vi "3DS Scene Mode.vi"(8 "error in (no error)":errorcluster, 10 "Draw Style:Mode":T1(ring), 11 "SceneObject in":refnum<vi>) -> (0 "error out":errorcluster, 3 "SceneObject out":refnum<vi>)   [LabVIEW 2026, in "3D utilities.lvlib"]
uses:
  3D utilities.lvlib
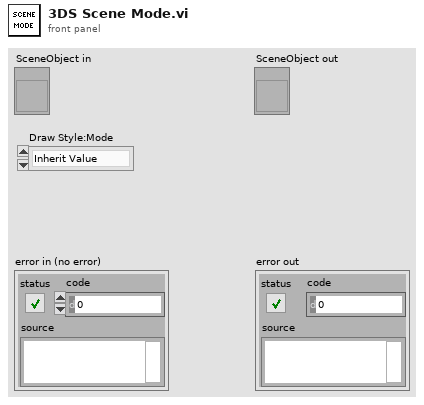
[diagram p1: front panel]
types:
  T1 = enum16{"Inherit Value", "Points", "Wireframe", "Polygons"}
  T2 = enum16{"Inherit Value", "No Culling", "Cull Back Face", "Cull Front Face", "Cull Both Faces"}
  T3 = enum16{"Zero", "One", "Destination Color", "One Minus Destination Color", "Source Alpha", "One Minus Source Alpha", "Destination Alpha", "One Minus Destination Alpha", "Source Alpha Saturate"}
  T4 = enum16{"Zero", "One", "Source Color", "One Minus Source Color", "Source Alpha", "One Minus Source Alpha", "Destination Alpha", "One Minus Destination Alpha"}
  T5 = enum16{"Normal Bin", "Opaque Bin", "Transparent Bin"}
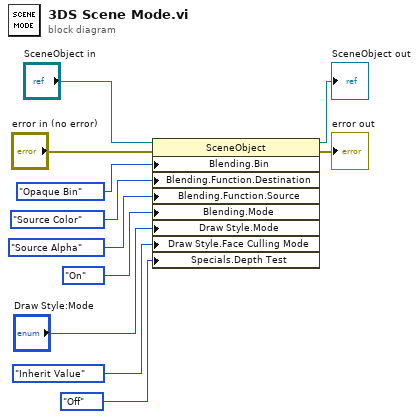
[diagram p0: block diagram]
diagram:
  n1 = property class="SceneObject"(reference="SceneObject in", error in="error in (no error)", "Blending.Bin"=T5."Opaque Bin" ("Blending:Bin"), "Blending.Function.Destination"=T4."Source Color" ("Blending:Function:Destination"), "Blending.Function.Source"=T3."Source Alpha" ("Blending:Function:Source"), "Blending.Mode"=enum16{"Inherit Value", "Off", "On"}."On" ("Blending:Mode"), "Draw Style.Mode"="Draw Style:Mode", "Draw Style.Face Culling Mode"=T2."Inherit Value" ("Draw Style:Face Culling Mode"), "Specials.Depth Test"=enum16{"Inherit Value", "Off", "On"}."Off" ("Specials:Depth Test")) -> (reference out=→"SceneObject out":refnum<vi>, error out=→"error out":errorcluster)
